vi "SP Convert Waveform to X-Y.vi"(1 "Waveform":cluster{"X0":dbl, "dX":dbl, "Y":dbl[]}) -> (0 "X-Y":cluster{"X":dbl[], "Y":dbl[]})   [LabVIEW 2011]
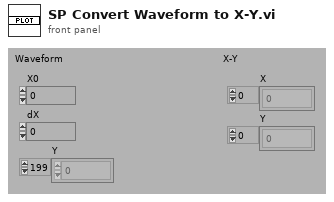
[diagram p1: front panel]
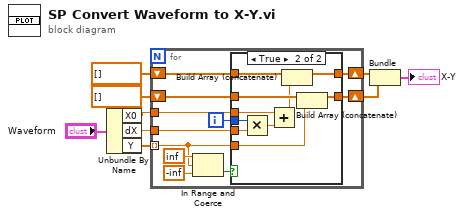
[diagram p0: block diagram]
diagram:
  n1 = Unbundle By Name("Waveform") -> ("X0"=w6:dbl, "dX"=w7:dbl, "Y"=w5:dbl[])
  n2 = for {
    tunnel: w7 -> [w15]
    tunnel: w6 -> [w16]
    tunnel: w5 -> [w11] mode=indexing
    shift-right: [w18] -> w1
    shift-left: dbl[] [] ("Y") -> [w19]
    shift-right: [w17] -> w2
    shift-left: dbl[] [] ("X") -> [w20]
    i -> [w14]
    n3 = In Range and Coerce(upper limit=inf, x=w11, lower limit=-inf) -> (In Range?=w10:bool)  [unwired: 1 out]
    n4 = case shown="True" w10 {
      tunnel: w20 -> [w21 w32]
      tunnel: w19 -> [w22 w30]
      tunnel: [w22 w29] -> w18
      tunnel: [w21 w31] -> w17
      tunnel: w16 -> [_ w27]
      tunnel: w15 -> [_ w24]
      tunnel: w14 -> [_ w25]
      tunnel: w11 -> [_ w23]
      frame False {
      }
      frame True {
        n5 = Multiply(x=w25, y=w24) -> (x*y=w28:dbl)
        n6 = Add(x=w27, y=w28) -> (x+y=w26:dbl)
        n7 = Build Array (concatenate)(w32, w26) -> (w31:dbl[])
        n8 = Build Array (concatenate)(w30, w23) -> (w29:dbl[])
      }
    }
  }
  n9 = Bundle("X"=w2, "Y"=w1) -> (→"X-Y":cluster{"X":dbl[], "Y":dbl[]})  [unwired: 1 out]
